vi "Create SimpleText.vi"(8 "error in (no error)":errorcluster, 10 "simpleText":string, 11 "ooDocument":refnum<class "ooDocument.lvclass">) -> (0 "error out":errorcluster, 2 "SimpleText":refnum<k24>, 3 "ooDocument out":refnum<class "ooDocument.lvclass">)   [LabVIEW 2009, in "ooDocument.lvclass"]
uses:
  ooDocument.lvclass
  C:/Projets/LAVAG/OpenOfficeRGT/AODL/DLLs/AODL.dll
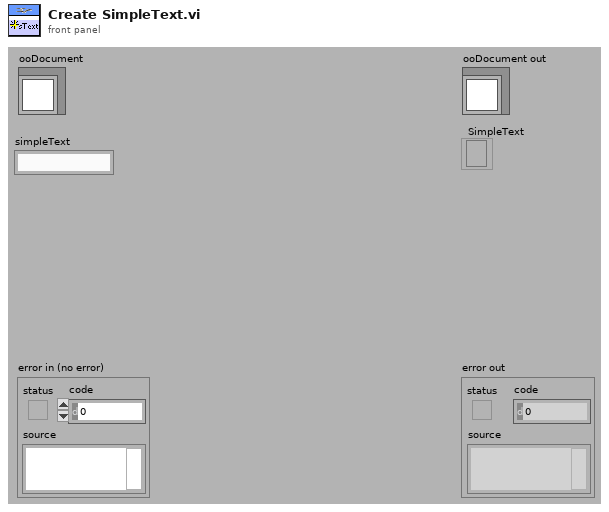
[diagram p1: front panel]
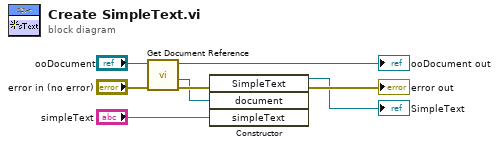
[diagram p0: block diagram]
diagram:
  n1 = call-dynamic "Get Document Reference.vi"("error in (no error)"="error in (no error)", "ooDocument in"="ooDocument") -> ("error out"=w2:errorcluster, "Document"=w1:refnum<k24>, "ooDocument out"=→"ooDocument out":refnum<class "ooDocument.lvclass">)  [unwired: 7 in]
  n2 = constructor class="SimpleText"(error in=w2, "document"=w1, "simpleText"="simpleText") -> (reference out=→"SimpleText":refnum<k24>, error out=→"error out":errorcluster)  [unwired: 2 in, 3 out]
